vi "RT Driver VI.vi"(7 "Operation":T1, 11 "Device Reference in":T2 format="%.0x") -> (0 "Error Code":i32)   [LabVIEW 2015, in "Protection and Counter Addon Engine.lvlib"]
uses:
  Protection and Counter Addon Engine.lvlib
  <vilib>/NI Veristand/Custom Device API/Custom Device Item Ref.ctl
  <vilib>/NI Veristand/Custom Device API/Hardware Interface Driver VI Operation.ctl
  <vilib>/NI/NIVS Inline Async API/_VS Inline Async API/VS Inline Async API/VS Inline Async API.lvclass
  Types/RT Async Engine Variables.ctl
  SubModules/Frame Protection Support/Source/Engine/Types/RT Frame Settings.ctl
  SubModules/Frame Protection Support/Source/Shared/Types/Exported Frame Type.ctl
  SubModules/Frame Protection Support/Source/Engine/Types/RT Protection Configuration.ctl
  SubModules/Frame Protection Support/Source/Shared/Types/Protection Type.ctl
  SubModules/Frame Protection Support/Source/Shared/Types/XNET Signal Configuration.ctl
  SubModules/Frame Protection Support/Source/Shared/Types/Exported Counter Settings.ctl
  SubModules/Frame Protection Support/Source/Shared/Types/Exported Event Trigger Type.ctl
  SubModules/Frame Protection Support/Source/Shared/Types/Exported Frame Settings.ctl
  SubModules/Frame Protection Support/Source/Shared/Types/Exported Protection Settings.ctl
  SubModules/Frame Protection Support/Source/Shared/Types/RT_Incoming_Signal_Info.ctl
  SubModules/Frame Protection Support/Source/Shared/Types/RT Exported Signal Settings.ctl
  Shared/Types/Exported.OnCompile.ctl
  Shared/Types/XNET Settings.ctl
  Shared/Types/986x.ctl
  SubModules/Frame Protection Support/Source/Shared/Types/Incoming Signal Info.ctl
  SubModules/Frame Protection Support/Source/Shared/Types/Exported Signal Settings.ctl
  <vilib>/NI/NIVS Inline Async API/_VS Inline Async API/VS Inline Async API/VS Inline Async API.lvclass/VS Inline Async API.ctl
  <vilib>/NI/NIVS Inline Async API/_Data Access Engine/Data Access Engine/Data Access Engine.lvclass/Data Access Engine.ctl
  <vilib>/NI/NIVS Inline Async API/_Data Access Engine/Access Type Classes/Write/Write.lvclass/Write.ctl
  <vilib>/NI/NIVS Inline Async API/_Data Access Engine/Access Type Classes/ReadWrite/ReadWrite.lvclass/ReadWrite.ctl
  <vilib>/NI/NIVS Inline Async API/_Data Access Engine/Access Type Classes/Read/Read.lvclass/Read.ctl
  <vilib>/NI/NIVS Inline Async API/_Data Access Engine/Data Access Engine/Methods/Data.Engine.Read Data from HW.vi
  <vilib>/NI/NIVS Inline Async API/_VS Inline Async API/Error Handling Process/SubVIs/Error.GetError.vi
  <vilib>/NI/NIVS Inline Async API/_Data Access Engine/Data Access Engine/Methods/Data.Engine.Write Data to HW.vi
  <vilib>/NI/NIVS Inline Async API/_Data Access Engine/Access Type Classes/ReadWrite/ReadWrite.EngineData.vi
  <vilib>/NI/NIVS Inline Async API/_Data Access Engine/Access Type Classes/Write/Write.EngineData.vi
  <vilib>/NI/NIVS Inline Async API/_Data Access Engine/Access Type Classes/Read/Read.EngineData.vi
  <vilib>/NI Veristand/Custom Device API/NI VeriStand - Get Channel Value by Data Reference.vi
  <vilib>/NI Veristand/Custom Device API/NI VeriStand - Set Channel Value by Data Reference.vi
  <vilib>/NI Veristand/Custom Device API/NI VeriStand - Get Channel Values by Block Data Reference.vi
  Shared/SubVIs/GUID Lookup.vi
  <vilib>/NI Veristand/Custom Device API/Get Item Property (Variant).vi
  <vilib>/NI Veristand/Custom Device API/Global Data Refs.vi
  <vilib>/NI VeriStand/Custom Device Tools/Custom Device Utility Library/Custom Device Utility Library.lvlib
  <vilib>/NI VeriStand/Custom Device API/Custom Device API.lvlib
  Shared/Protection and Counter Addon Shared.lvlib
  SubModules/Frame Protection Support/Source/Shared/Protection and Counter Support Shared.lvlib
  SubModules/Frame Protection Support/Source/Engine/Protection and Counter Support Engine.lvlib
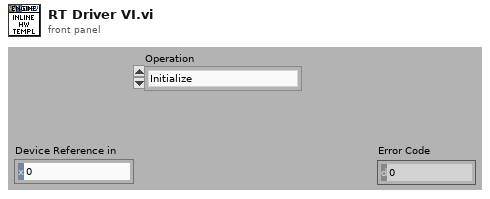
[diagram p1: front panel]
types:
  T1 = typedef "Custom Device API.lvlib/Hardware Interface Driver VI Operation.ctl" = enum16{"Initialize", "Start", "Read Data from HW", "Write Data to HW", "Close"}
  T2 = typedef "Custom Device API.lvlib/Custom Device Item Ref.ctl" = u64
  T3 = typedef "Protection and Counter Addon Engine.lvlib/RT Async Engine Variables.ctl" = cluster{"Priority":i32, "CAN Session":refnum<k21>, "Frame Count":i32, "Frames":T4[], "FPGA Session":u32, "Incoming Frame Session":refnum<k21>, "Incoming Session Invalid":bool, "Incoming Frames":T11[], "Signal Values":dbl[], "Incoming Signal Info":T13}
  T4 = typedef "Protection and Counter Support Engine.lvlib/RT Frame Settings.ctl" = cluster{"Type":T5, "Frame ID":u32, "Payload Length":u32, "VS Offset":i32, "VS Length":i32, "Frame Conversion":refnum<k21>, "Frame.PrevData":dbl[], "Generation Period":u32, "Time Since Last Generation":u32, "Generation Iterations":u32, "Generation Counter":u32, "Has Protection?":bool, "Protection Configurations":T6[], "Has Counter?":bool, "Counter Configurations":T9[], "Has Disable?":bool, "Disable VS Index":i32, "Transmit Trigger":T10, "Trigger VS Index":i32}
  T5 = typedef "Protection and Counter Support Shared.lvlib/Exported Frame Type.ctl" = enum16{"Periodic", "Event", "Periodic/Event"}
  T6 = typedef "Protection and Counter Support Engine.lvlib/RT Protection Configuration.ctl" = cluster{"Protection Frame Index":i32, "Protection Type":T7, "Data Indeces":i32[], "Initialized Data Array":dbl[], "Check Sum Conversion":refnum<k21>, "CRC Channels":T8[], "Protection VS Index":i32}
  T7 = typedef "Protection and Counter Support Shared.lvlib/Protection Type.ctl" = enum16{"Arb ID + Bytes Checksum with Inversion", "Arb ID + Bytes CRC with Inversion", "Reversed Raw Signal Checksum with Inversion"}
  T8 = typedef "Protection and Counter Support Shared.lvlib/XNET Signal Configuration.ctl" = cluster{"Start Bit":i32, "Name":string, "Number of bits":i32, "Scale":dbl, "Offset":dbl, "Data Type":u32}
  T9 = typedef "Protection and Counter Support Shared.lvlib/Exported Counter Settings.ctl" = cluster{"Counter Frame Index":i32, "Max Count":dbl, "Counter VS Index":i32}
  T10 = typedef "Protection and Counter Support Shared.lvlib/Exported Event Trigger Type.ctl" = enum16{"Channel value change", "Trigger channel (not zero)", "Channel value change or trigger channel (not zero)", "Trigger channel (any value change)", "Channel value change or trigger channel (any value change)"}
  T11 = typedef "Protection and Counter Support Shared.lvlib/Exported Frame Settings.ctl" = cluster{"Type":T5, "Frame ID":u32, "Payload Length":u32, "Signal XNET Paths":string[], "Frame.PrevData":dbl[], "VS Offset":i32, "VS Length":i32, "Generation Period":u32, "Has Protection?":bool, "Protection Configurations":T12[], "Has Counter":bool, "Counter Configurations":T9[], "Has Disable?":bool, "Disable VS Index":i32, "Transmit Trigger":T10, "Trigger VS Index":i32}
  T12 = typedef "Protection and Counter Support Shared.lvlib/Exported Protection Settings.ctl" = cluster{"Protection Frame Index":i32, "Protection Type":T7, "Data Indeces":i32[], "Initialized Data Array":dbl[], "Protection Signal XNET Paths":string[], "CRC Channels":T8[], "Protection VS Update Index":i32}
  T13 = typedef "Protection and Counter Support Shared.lvlib/RT_Incoming_Signal_Info.ctl" = cluster{"Signal.PrevData":dbl[], "Signal Names":string[], "Signal Settings Out":T14[]}
  T14 = typedef "Protection and Counter Support Shared.lvlib/RT Exported Signal Settings.ctl" = cluster{"Is Protection":bool, "Is Counter":bool, "Signal Name":string, "Counter Configuration":T9, "Valid_Sig_Ref_Index":i32, "Frame ID":u32, "Payload Length":u32, "Protection Configuration":T6}
  T15 = cluster{"Process":refnum<class "VS Inline Async API.lvclass">, "Device.Error":errorcluster, "RT Configuration":T3}
  T16 = typedef "Protection and Counter Addon Shared.lvlib/Exported.OnCompile.ctl" = cluster{"XNET Settings":T17, "Frames":T11[], "986x Support":T18, "Incoming Frames":T11[], "Incoming Signal Info":T19}
  T17 = typedef "Protection and Counter Addon Shared.lvlib/XNET Settings.ctl" = cluster{"Database":refnum<k21>, "Cluster":refnum<k21>, "Port":string, "Baud rate [Bd]":u64, "Termination":u32, "CAN I/O Mode":u32, "FD Baud rate [Bd]":u64, "Priority":i32, "Use Legacy":bool}
  T18 = typedef "Protection and Counter Addon Shared.lvlib/986x.ctl" = cluster{"Enable":bool, "RIO Device":string, "Bitfile":path}
  T19 = typedef "Protection and Counter Support Shared.lvlib/Incoming Signal Info.ctl" = cluster{"Signal Settings Out":T20[], "Signal.PrevData":dbl[], "Signal Names":string[]}
  T20 = typedef "Protection and Counter Support Shared.lvlib/Exported Signal Settings.ctl" = cluster{"Is Protection":bool, "Is Counter":bool, "Signal Name":string, "Counter Configuration":T9, "Protection Configuration":T12, "Valid_Sig_Ref_Index":i32, "Frame ID":u32, "Payload Length":u32}
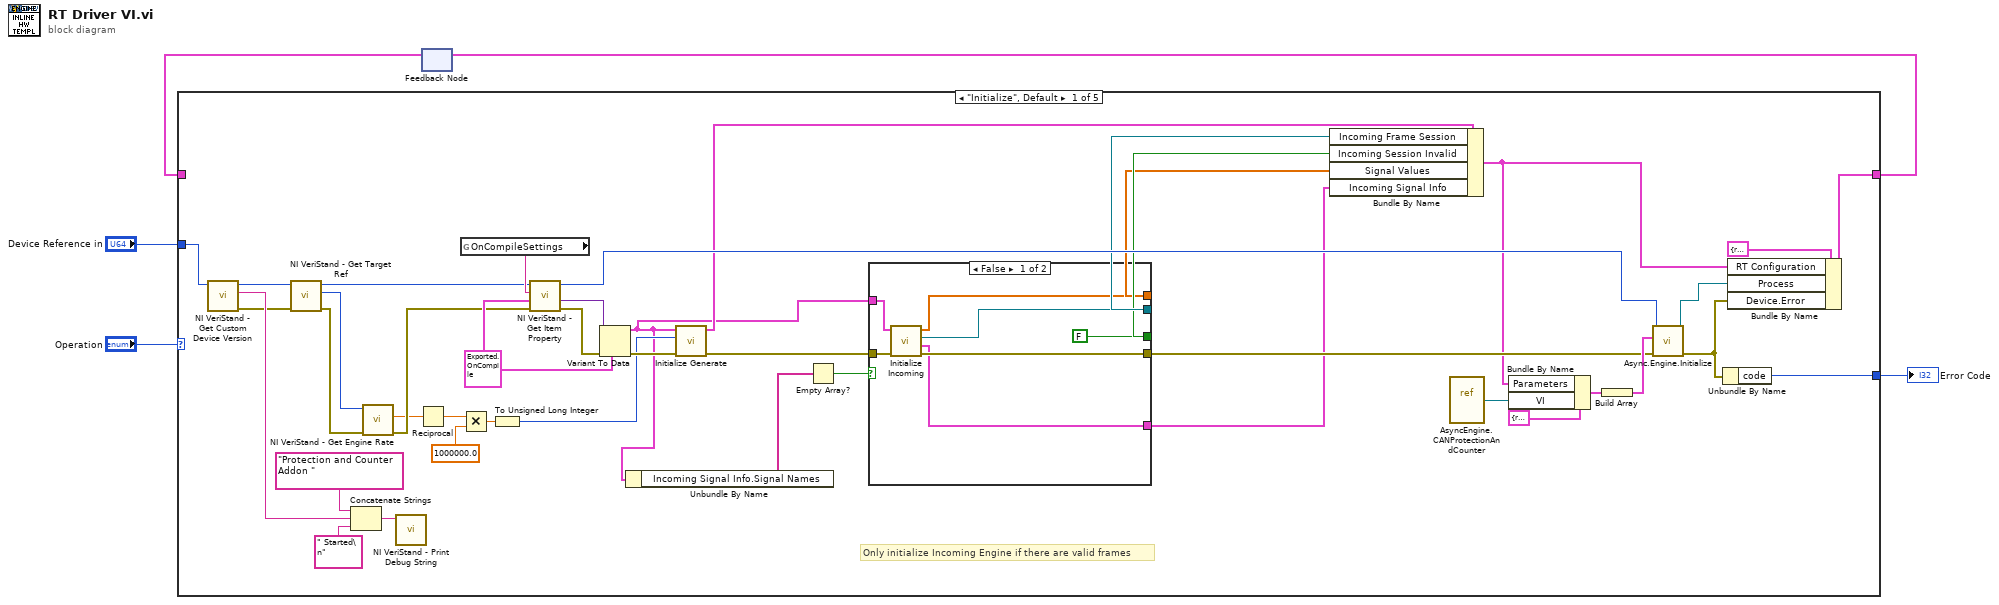
[diagram p0: block diagram]
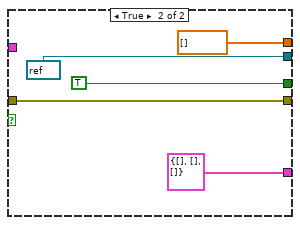
[diagram p2: hidden frame]
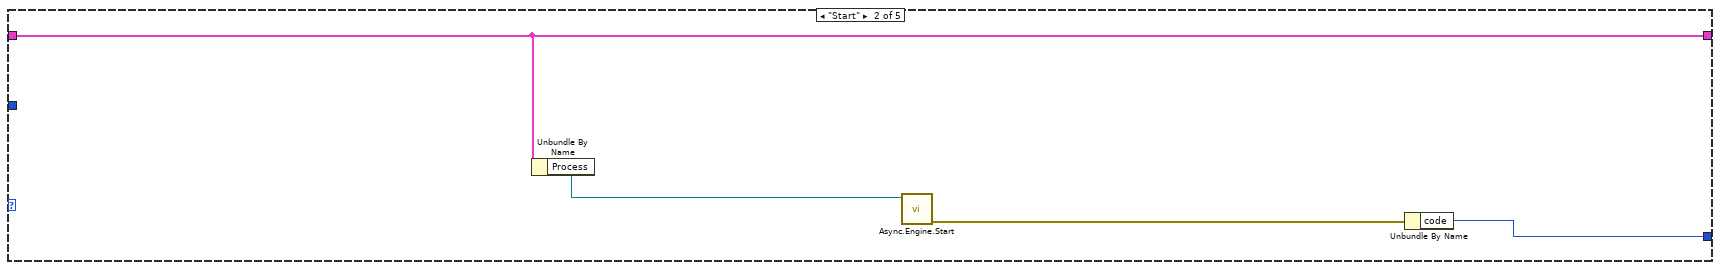
[diagram p3: hidden frame]
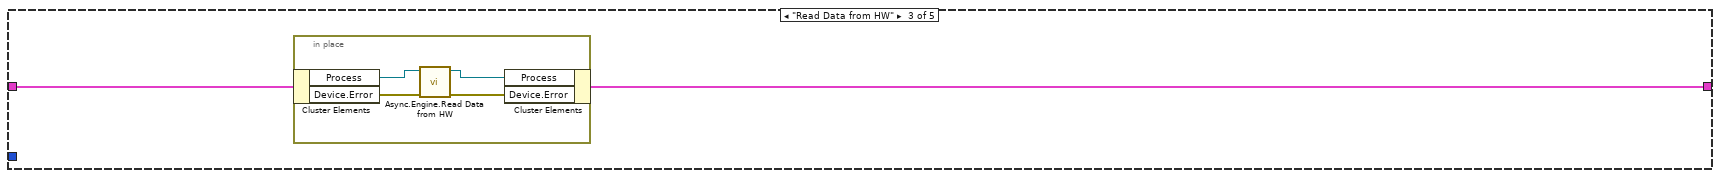
[diagram p4: hidden frame]
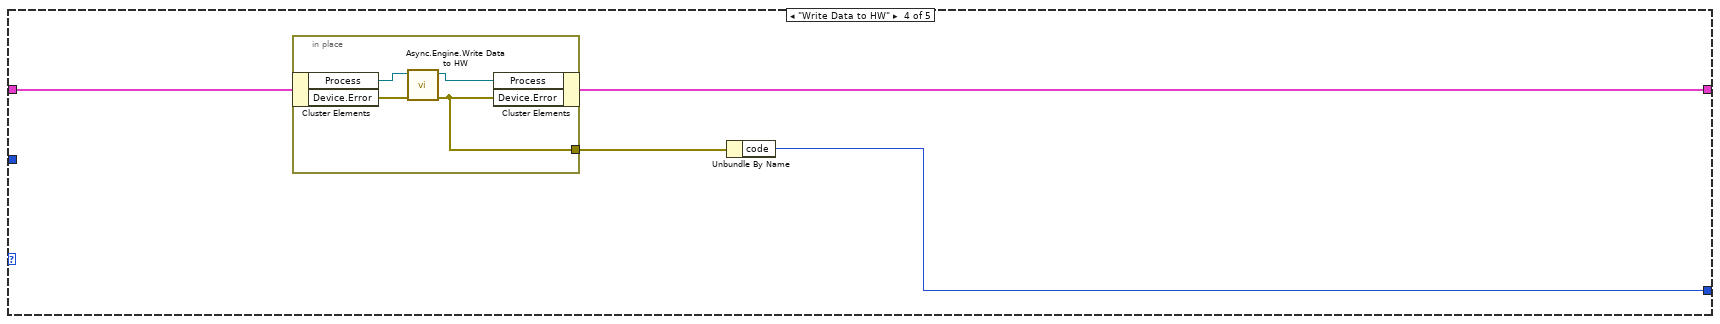
[diagram p5: hidden frame]
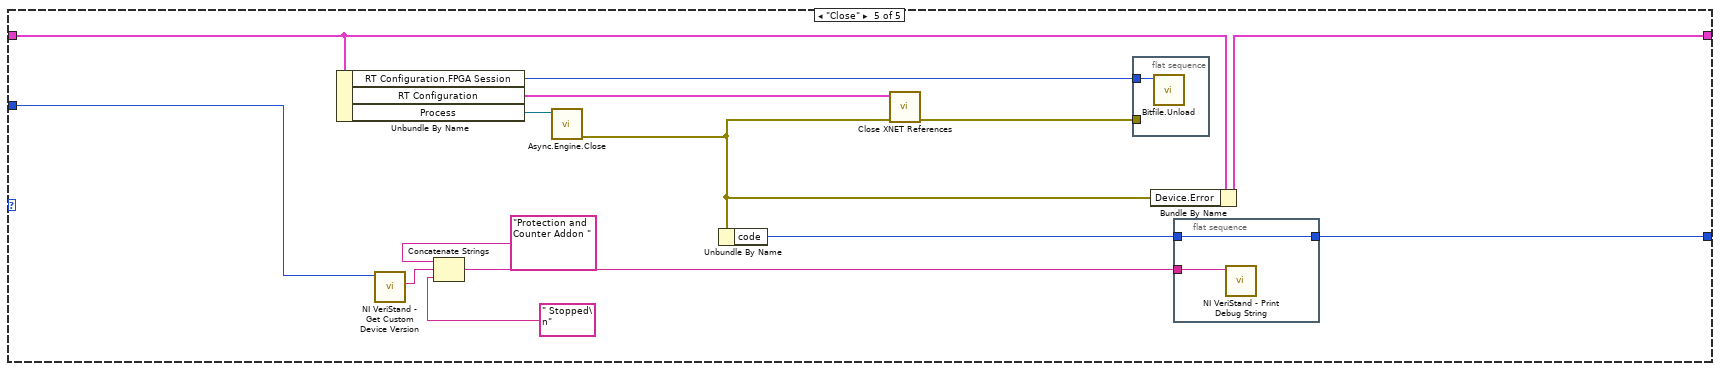
[diagram p6: hidden frame]
diagram:
  n1 = feedback #1() -> (w3:T15)  [unwired: 1 out]
  n2 = case shown="\"Initialize\", Default" "Operation" {
    tunnel: [w46 w60 w64 w73 w91] -> w4
    tunnel: w3 -> [_ w60 w65 w72 w83]
    tunnel: [w47 w63 _ w70 w84] -> w2
    tunnel: "Device Reference in" -> [w43 _ _ _ w87]
    frame "Initialize", Default {
      w30 = T16 {"XNET Settings"={"Database"="", "Cluster"="", "Port"="", "Baud rate [Bd]"=500000, "Termination"=1, "CAN I/O Mode"=0, "FD Baud rate [Bd]"=500000, "Priority"=100, "Use Legacy"=FALSE}, "Frames"=[], "986x Support"={"Enable"=FALSE, "RIO Device"="", "Bitfile"=path ""}, "Incoming Frames"=[], "Incoming Signal Info"={"Signal Settings Out"=[], "Signal.PrevData"=[], "Signal Names"=[]}} ("Cluster")
      # "Only initialize Incoming Engine if there are valid frames"
      n3 = call <vilib>:"NI VeriStand - Get Custom Device Version.vi"("Device Ref in"=w43) -> ("error out"=w24:errorcluster, "Value"=w42:string, "Device Ref out"=w33:T2)  [unwired: 8 in]
      n4 = call <vilib>:"NI VeriStand - Get Target Ref.vi"("error in"=w24, "Item Ref in"=w33) -> ("error out"=w23:errorcluster, "Target Ref"=w25:T2, "Item Ref out"=w26:T2)  [unwired: 6 in, 1 out]
      n5 = Concatenate Strings("Protection and Counter Addon " ("Debug String"), w42, " Started\n" ("string")) -> (w44:string)
      n6 = call <vilib>:"NI VeriStand - Get Engine Rate.vi"("error in (no error)"=w23, "Item Ref in"=w25) -> ("error out"=w22:errorcluster, "Rate (Hz)"=w21:dbl)  [unwired: 7 in, 1 out]
      n7 = call <vilib>:"NI VeriStand - Print Debug String.vi"("Message"=w44) -> ()  [unwired: 10 in, 1 out]
      n8 = Reciprocal(x=w21) -> (1/x=w20:dbl)
      n9 = global read "GUID Lookup.vi" "OnCompileSettings"() -> (w34:string)
      n10 = Multiply(x=w20, y=1000000.0) -> (x*y=w18:dbl)
      n11 = To Unsigned Long Integer(number=w18) -> (unsigned 32bit integer=w17:u32)
      n12 = call-poly <vilib>:"NI VeriStand - Get Item Property.vi"("error in (no error)"=w22, "Default Value"=w30, "Property Name"=w34, "Item Ref in"=w26) -> ("error out"=w31:errorcluster, "Value"=w32:variant, "Item Ref out"=w29:T2)  [unwired: 4 in, 1 out]
      n13 = Variant To Data(error in=w31, type=w30, Variant=w32) -> (data=w11:T16, error out=w28:errorcluster)
      n14 = Unbundle By Name(w11) -> ("Incoming Signal Info.Signal Names"=w10:string[])
      n15 = call "Initialize Generate.vi"("error in (no error)"=w28, "PCL (usec)"=w17, "OnCompile Variables"=w11) -> ("error out"=w16:errorcluster, "RT Configuration"=w14:T3)  [unwired: 7 in]
      n16 = Empty Array?(array=w10) -> (empty?=w9:bool)
      n17 = case shown="False" w9 {
        tunnel: w16 -> [w54 w59]
        tunnel: [w53 w59] -> w15
        tunnel: [w52 refnum<k21> refnum ("Incoming CAN Session")] -> w12
        tunnel: w11 -> [w51 _]
        tunnel: [FALSE TRUE] -> w8
        tunnel: [w49 dbl[] [] ("Signal Values")] -> w7
        tunnel: [w48 T13 {"Signal.PrevData"=[], "Signal Names"=[], "Signal Settings Out"=[]} ("RT Incoming Signal Info")] -> w6
        frame False {
          n18 = call "Initialize Incoming.vi"("error in (no error)"=w54, "OnCompile Variables"=w51) -> ("error out"=w53:errorcluster, "RT Incoming Signal Info"=w48:T13, "Incoming CAN Session"=w52:refnum<k21>, "Signal Values"=w49:dbl[])  [unwired: 6 in]
        }
        frame True {
        }
      }
      n19 = Bundle By Name(cluster=w14, "Incoming Frame Session"=w12, "Incoming Session Invalid"=w8, "Signal Values"=w7, "Incoming Signal Info"=w6) -> (w13:T3)
      n20 = vi-ref "AsyncEngine.CANProtectionAndCounter.vi"() -> (w27:refnum<vi>)
      n21 = Bundle By Name(cluster=cluster{"VI":refnum<vi>, "Parameters":variant} {"VI"=refnum, "Parameters"=variant} ("Process"), "Parameters"=w13, "VI"=w27) -> (w37:cluster{"VI":refnum<vi>, "Parameters":variant})
      n22 = Build Array(w37) -> (w36:cluster{"VI":refnum<vi>, "Parameters":variant}[])
      n23 = call <vilib>:"Async.Engine.Initialize.vi"("error in (no error)"=w15, "Processes"=w36, "Custom Device Ref"=w29) -> ("error out"=w40:errorcluster, "Async"=w39:refnum<class "VS Inline Async API.lvclass">)  [unwired: 7 in]
      n24 = Unbundle By Name(w40) -> ("code"=w47:i32)
      n25 = Bundle By Name(cluster=T15 {"Process"=refnum, "Device.Error"={"status"=FALSE, "code"=0, "source"=""}, "RT Configuration"={"Priority"=100, "CAN Session"="", "Frame Count"=0, "Frames"=[], "FPGA Session"=0, "Incoming Frame Session"="", "Incoming Session Invalid"=FALSE, "Incoming Frames"=[], "Signal Values"=[], "Incoming Signal Info"={"Signal.PrevData"=[], "Signal Names"=[], "Signal Settings Out"=[]}}} ("input cluster"), "RT Configuration"=w13, "Process"=w39, "Device.Error"=w40) -> (w46:T15)
    }
    frame "Start" {
      n26 = Unbundle By Name(w60) -> ("Process"=w62:refnum<class "VS Inline Async API.lvclass">)
      n27 = call <vilib>:"Async.Engine.Start.vi"("VS Inline Async API in"=w62) -> ("error out"=w61:errorcluster)  [unwired: 9 in, 1 out]
      n28 = Unbundle By Name(w61) -> ("code"=w63:i32)
    }
    frame "Read Data from HW" {
      n29 = in-place {
        n30 = in-place-cluster #2(w65) -> ("Process"=w69:refnum<class "VS Inline Async API.lvclass">, "Device.Error"=w67:errorcluster)
        n31 = call <vilib>:"Async.Engine.Read Data from HW.vi"("error in"=w67, "Async in"=w69) -> ("error out"=w66:errorcluster, "Async out"=w68:refnum<class "VS Inline Async API.lvclass">)  [unwired: 8 in]
        n32 = in-place-cluster #2("Process"=w68, "Device.Error"=w66) -> (w64:T15)
      }
    }
    frame "Write Data to HW" {
      n33 = in-place {
        in-place-border: [w74] -> w71
        n34 = in-place-cluster #3(w72) -> ("Process"=w76:refnum<class "VS Inline Async API.lvclass">, "Device.Error"=w77:errorcluster)
        n35 = call <vilib>:"Async.Engine.Write Data to HW.vi"("error in (no error)"=w77, "VS Inline Async API in"=w76) -> ("error out"=w74:errorcluster, "VS Inline Async API out"=w75:refnum<class "VS Inline Async API.lvclass">)  [unwired: 8 in]
        n36 = in-place-cluster #3("Process"=w75, "Device.Error"=w74) -> (w73:T15)
      }
      n37 = Unbundle By Name(w71) -> ("code"=w70:i32)
    }
    frame "Close" {
      n38 = Unbundle By Name(w83) -> ("RT Configuration.FPGA Session"=w79:u32, "RT Configuration"=w81:T3, "Process"=w82:refnum<class "VS Inline Async API.lvclass">)
      n39 = call <vilib>:"NI VeriStand - Get Custom Device Version.vi"("Device Ref in"=w87) -> ("Value"=w90:string)  [unwired: 8 in, 2 out]
      n40 = Concatenate Strings("Protection and Counter Addon " ("Debug String"), w90, " Stopped\n" ("Debug String")) -> (w86:string)
      n41 = call <vilib>:"Async.Engine.Close.vi"("Async in"=w82) -> ("error out"=w80:errorcluster)  [unwired: 9 in, 1 out]
      n42 = Unbundle By Name(w80) -> ("code"=w85:i32)
      n43 = call "Close XNET References.vi"("error in (no error)"=w80, "RT Configuration"=w81) -> ("error out"=w78:errorcluster)  [unwired: 9 in]
      n44 = flat-sequence {
        tunnel: w79 -> [w92]
        tunnel: w78 -> [_]
        frame #0 {
          n45 = call "Bitfile.Unload.vi"("Session"=w92) -> ()  [unwired: 11 in]
        }
      }
      n46 = Bundle By Name(cluster=w83, "Device.Error"=w80) -> (w91:T15)
      n47 = flat-sequence {
        tunnel: w86 -> [w94]
        tunnel: [w93] -> w84
        tunnel: w85 -> [w93]
        frame #0 {
          n48 = call <vilib>:"NI VeriStand - Print Debug String.vi"("Message"=w94) -> ()  [unwired: 10 in, 1 out]
        }
      }
    }
  }
  "Error Code" <- w2
  n49 = feedback-in #1(w4) -> ()
